vi "Panel.vi"(11 "SimpleGraphEditorPanel in":refnum<class "SimpleGraphEditorPanel.lvclass">) -> ()   [LabVIEW 2020, in "VolatusGUIControls.lvlib" / "SimpleGraphEditorPanel.lvclass"]
uses:
  SimpleGraphEditorPanel.lvclass
  C:/dev/lv20CE/relink/volatus-gui-controls/VolatusGUIEditorCore/ElementEditorPanel/ElementEditorPanel.lvclass
  C:/dev/lv20CE/relink/lv-oopanel/OOPanel/Panel/Panel.lvclass
  lv-oopanel/OOPanel/Panel/Basic UI State.ctl
  SimpleGraphEditorPanel.lvclass/SimpleGraphEditorPanel.ctl
  lv-autocomplete/AutoComplete/Shared Options/Shared Options.lvclass/Shared Options.ctl
  lv-oopanel/OOPanel/Panel/Panel.lvclass
  lv-oopanel/OOPanel/OOPanel.lvlib
  VolatusGUIEditorCore/ElementEditorPanel/ElementEditorPanel.lvclass
  VolatusGUIEditorCore/VolatusGUIEditorCore.lvlib
  C:/dev/lv20CE/relink/volatus-gui-controls/VolatusGUIControls/SimpleGraphEditorPanel/SimpleGraphEditorPanel.lvclass
panel:
  in  "Legend Scrollbar":bool
  in  "Plot Visibility Checkbox":bool
  in  "Show Legend":bool
  in  "History Minutes":dbl
  in  "Scales":bool
  in  "Channels":bool
  in  "Top":i32
  in  "Left":i32
  in  "Height":u16
  in  "Width":u16
  in  "Label Text Color":u32(colorbox) caption="Color"
  in  "Label Visible":bool caption="Visible"
  in  "Label":string
  # "Label"
  # "Assumes 10Hz published data"
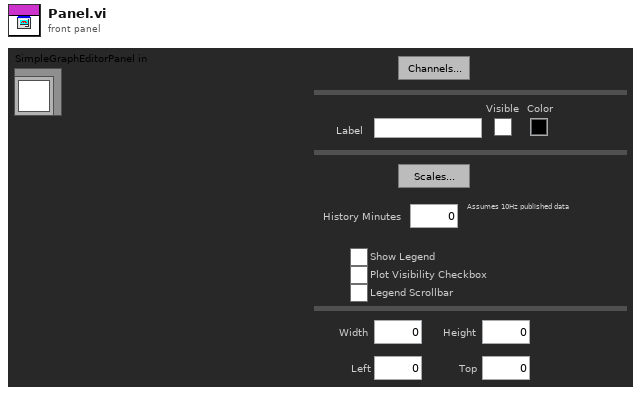
[diagram p1: front panel]
types:
  T1 = typedef "OOPanel.lvlib/Panel.lvclass/Basic UI State.ctl" = enum16{"Init", "Run", "Close"}
  T2 = typedef "VolatusGUIEditorCore.lvlib/ElementEditorPanel.lvclass/Incoming Events.ctl" = cluster{"Update Control":refnum<user-event>}
  T3 = typedef "OOPanel.lvlib/Panel.lvclass/Panel Events.ctl" = cluster{"Visbility":refnum<user-event>, "Close":refnum<user-event>}
  T4 = typedef "VolatusGUIControls.lvlib/SimpleGraphEditorPanel.lvclass/Props.ctl" = cluster{"JSON Props":T5, "Label":T6, "Position":T7, "Width":u16, "Height":u16, "Plot Legend":T8}
  T5 = typedef "VolatusGUIControls.lvlib/SimpleGraphEditorPanel.lvclass/JSON Props.ctl" = cluster{"Channels":string[], "Buffer_Length":i32, "Redraw_Period_s":dbl, "Duration_s":i32}
  T6 = typedef "VolatusGUIEditorCore.lvlib/Label Props.ctl" = cluster{"Text":string, "Text Color":u32, "Visible":bool}
  T7 = typedef "VolatusGUIEditorCore.lvlib/Position Props.ctl" = cluster{"Left":i32, "Top":i32}
  T8 = typedef "VolatusGUIEditorCore.lvlib/Plot Legend Props.ctl" = cluster{"Visible":bool, "Plot Visibility":bool, "Scrollbar":bool}
  T9 = typedef "OOPanel.lvlib/Visibility State.ctl" = enum16{"Idle", "Closed", "Hidden", "Visible", "Subpanel", "Hidden Subpanel"}
  T10 = cluster{"Label":string, "Label Text Color":u32, "Label Visible":bool}
  T11 = cluster{"Show Legend":bool, "Plot Visibility Checkbox":bool, "Legend Scrollbar":bool}
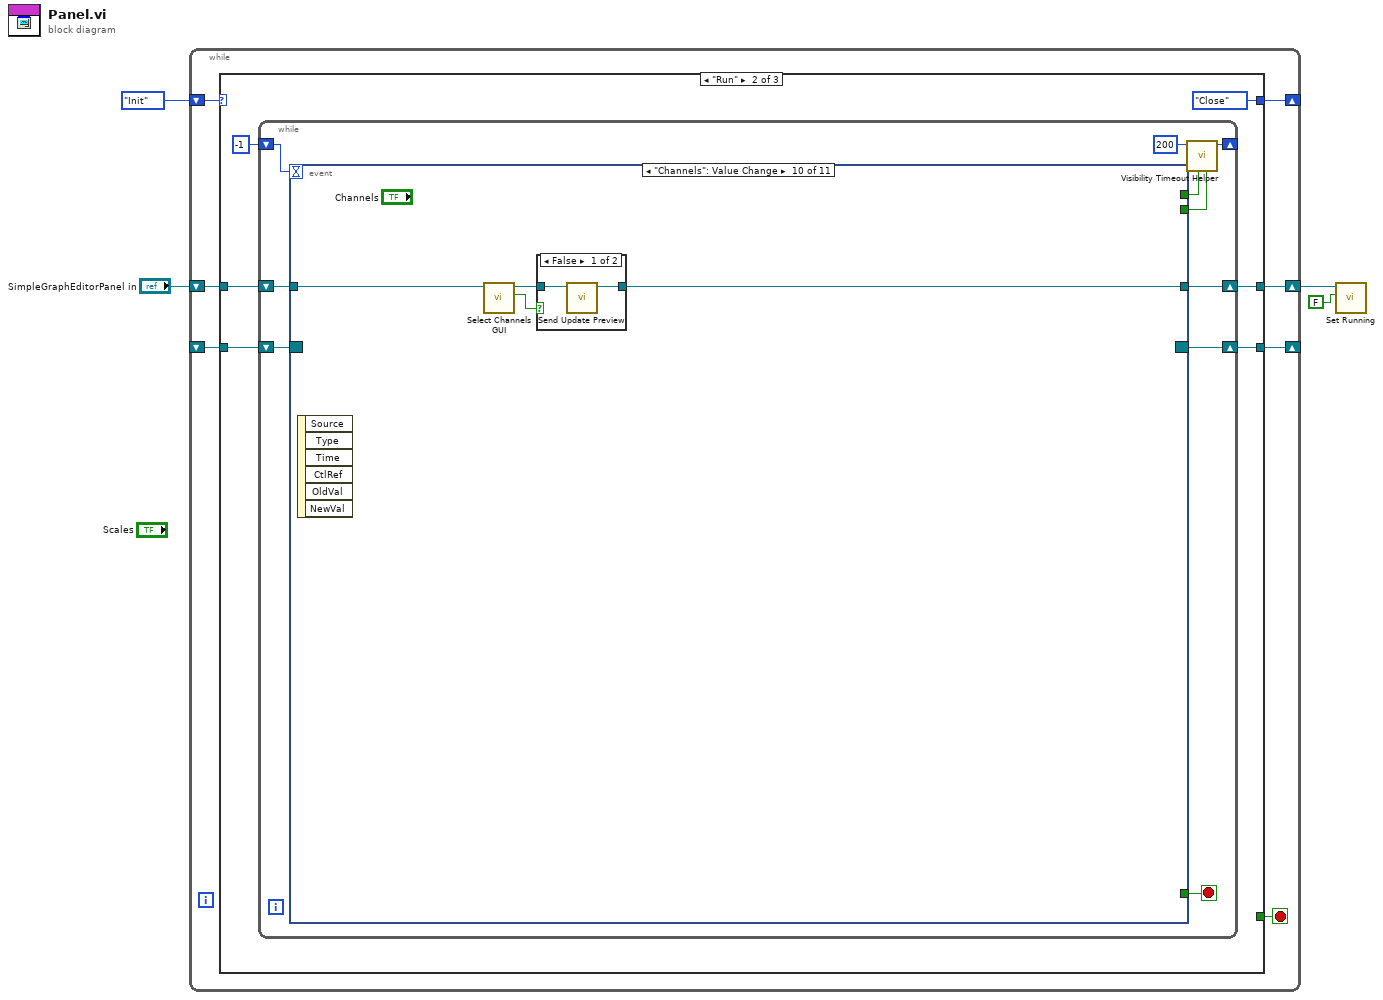
[diagram p0: block diagram]
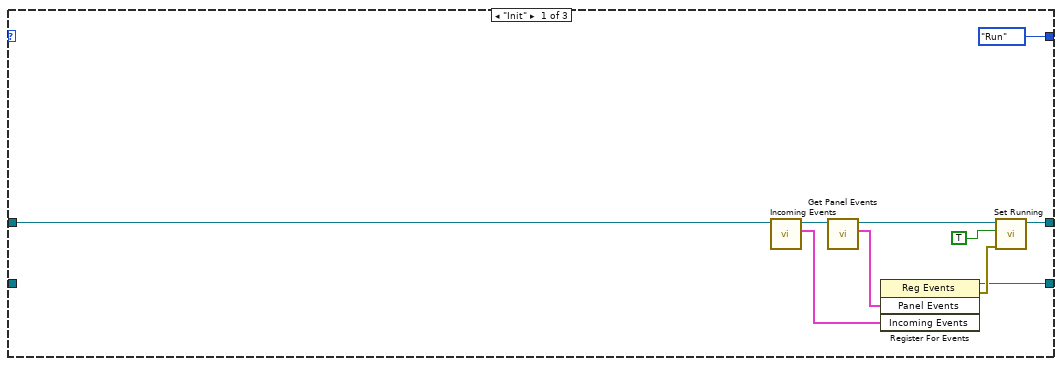
[diagram p2: hidden frame]
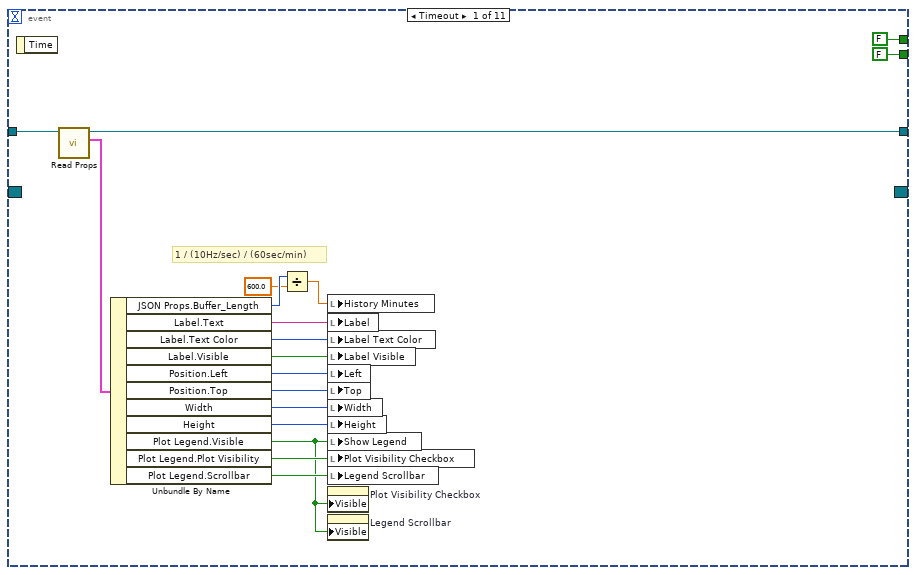
[diagram p3: hidden frame]
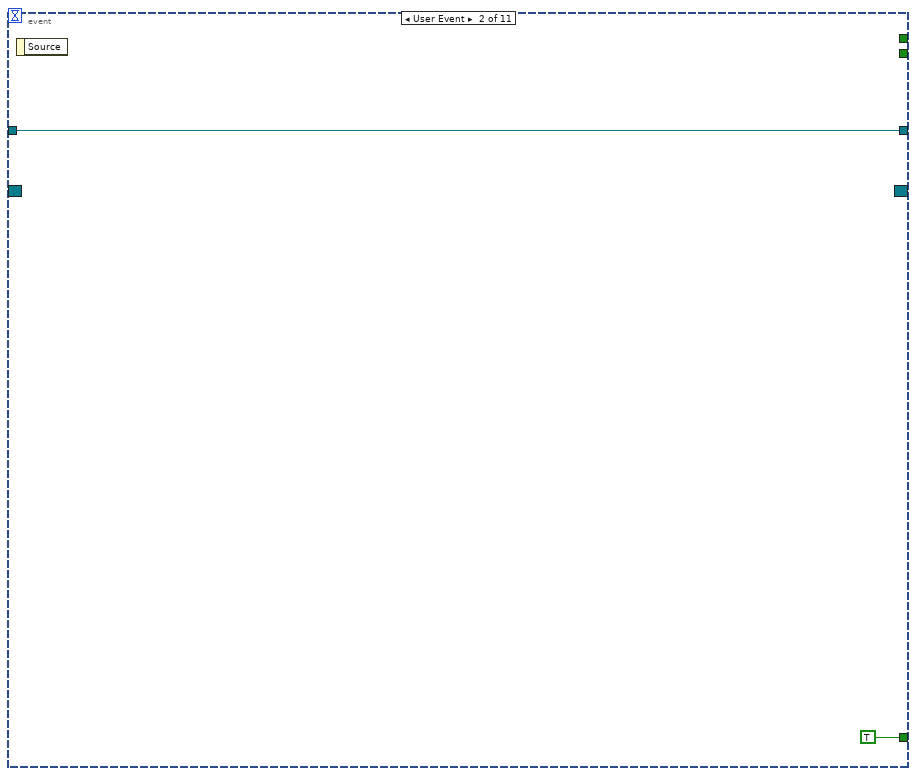
[diagram p4: hidden frame]
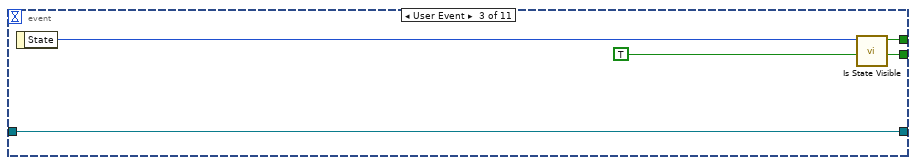
[diagram p5: hidden frame]
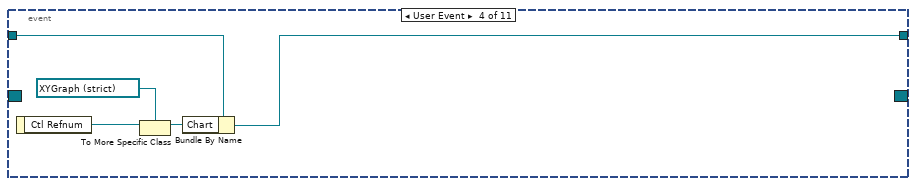
[diagram p6: hidden frame]
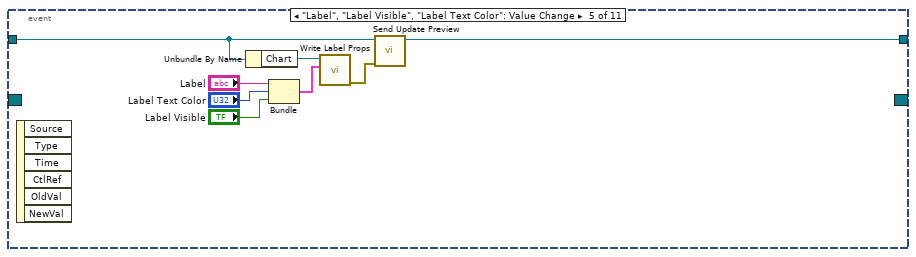
[diagram p7: hidden frame]
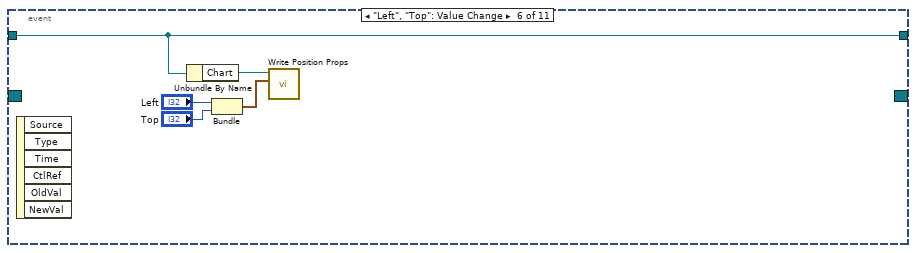
[diagram p8: hidden frame]
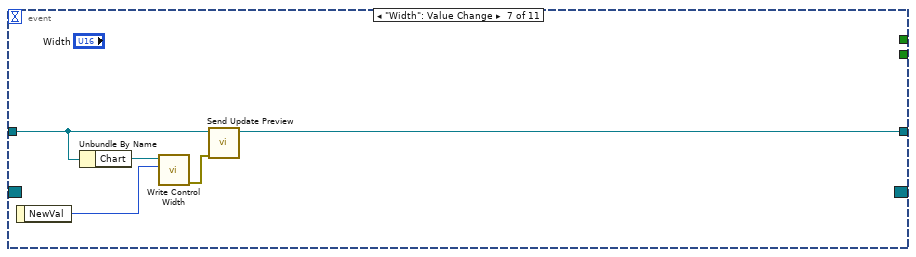
[diagram p9: hidden frame]
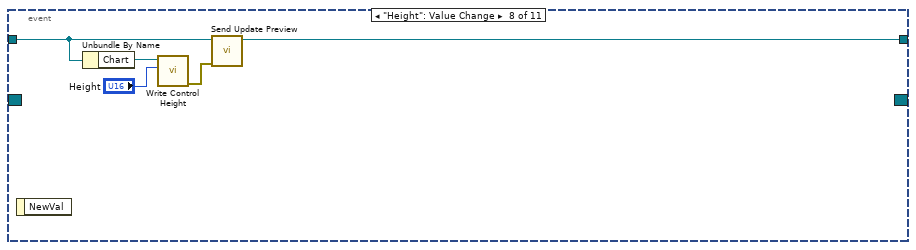
[diagram p10: hidden frame]
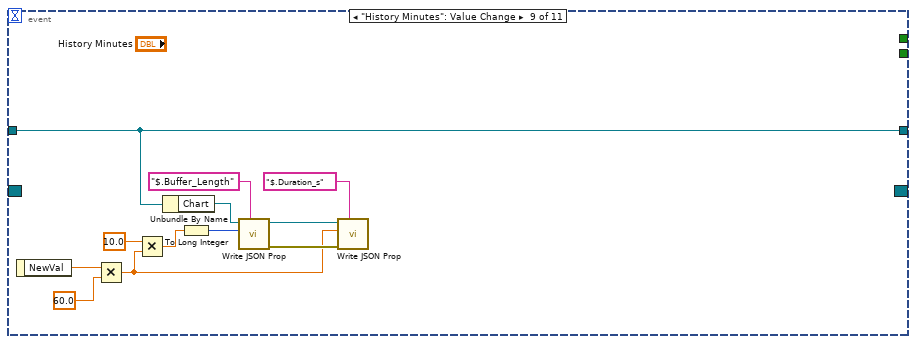
[diagram p11: hidden frame]
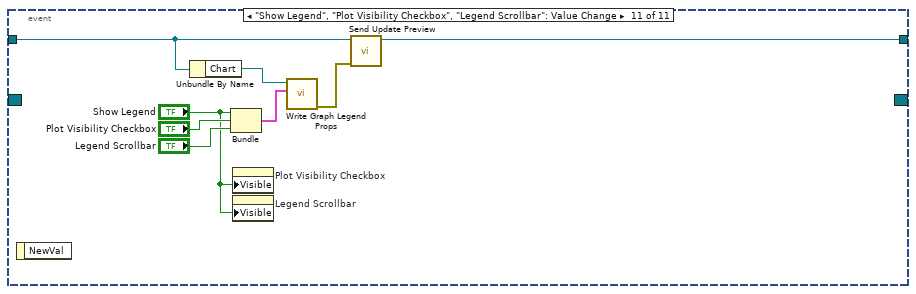
[diagram p13: hidden frame]
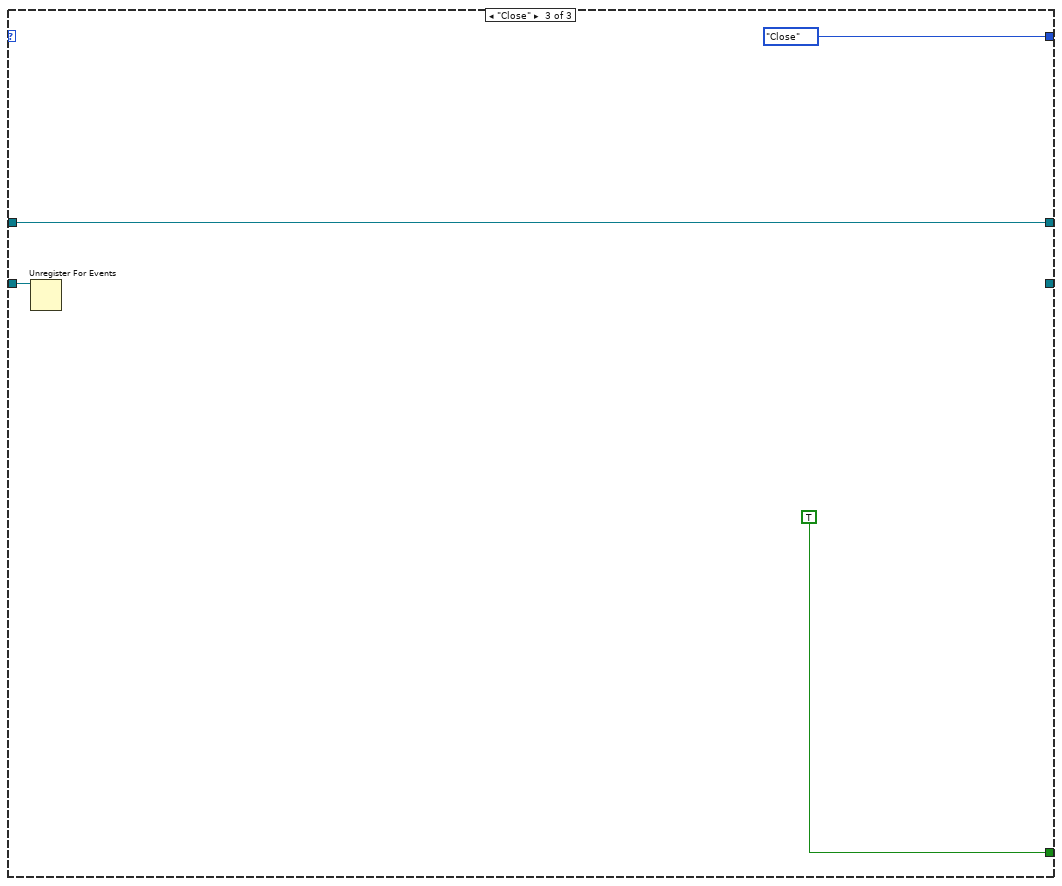
[diagram p14: hidden frame]
diagram:
  n1 = while {
    shift-right: [w10] -> _
    shift-left: _ -> [w11]
    shift-right: [w8] -> _
    shift-left: Basic_UI_State."Init" ("Basic UI State") -> [w9]
    shift-right: [w6] -> w4
    shift-left: "SimpleGraphEditorPanel in" -> [w5]
    stop <- w7 stop-if-true
    n2 = case shown="\"Run\"" w9 {
      tunnel: w11 -> [_ w27 w118]
      tunnel: [w18 w25 _] -> w10
      tunnel: [Basic_UI_State."Run" ("Basic UI State") Basic_UI_State."Close" ("Basic UI State") Basic_UI_State."Close" ("Basic UI State")] -> w8
      tunnel: [_ _ TRUE] -> w7
      tunnel: [w17 w22 w117] -> w6
      tunnel: w5 -> [w16 w23 w117]
      frame "Init" {
        n3 = call "Incoming Events.vi"("ElementEditorPanel in"=w16) -> ("Incoming Events"=w12:T2, "ElementEditorPanel out"=w13:refnum<class "SimpleGraphEditorPanel.lvclass">)  [unwired: 9 in]
        n4 = call "Get Panel Events.vi"("Panel in"=w13) -> ("Panel Events"=w14:T3, "Panel out"=w15:refnum<class "SimpleGraphEditorPanel.lvclass">)  [unwired: 8 in, 1 out]
        n5 = register-events(w14, w12) -> (reference out=w18:refnum<event-registration>, error out=w20:errorcluster)  [unwired: 2 in]
        n6 = call "Set Running.vi"("error in (no error)"=w20, "Running"=TRUE, "Panel in"=w15) -> ("Panel out"=w17:refnum<class "SimpleGraphEditorPanel.lvclass">)  [unwired: 7 in, 1 out]
      }
      frame "Run" {
        n7 = while {
          shift-right: [w33] -> w25
          shift-left: w27 -> [w34]
          shift-right: [w36] -> _
          shift-left: -1 ("Timeout") -> [w35]
          shift-right: [w28] -> w22
          shift-left: w23 -> [w29]
          stop <- w30 stop-if-true
          n8 = event shown="[9] \"Channels\": Value Change" {
            selector: w34 -> [_ _ _ _ _ _ _ _ _ _ _]
            dyn-events: [_ _ _ _ _ _ _ _ _ _ _] -> w33
            timeout: w35 -> [_ _ _ _ _ _ _ _ _ _ _]
            tunnel: [FALSE _ w60 _ _ _ _ _ _ _ _] -> w32
            tunnel: [FALSE _ TRUE _ _ _ _ _ _ _ _] -> w31
            tunnel: [_ TRUE _ _ _ _ _ _ _ _ _] -> w30
            tunnel: w29 -> [w53 w56 w58 w66 w72 w76 w84 w88 w97 w102 w116]
            tunnel: [w52 w56 w58 w64 w68 w76 w81 w86 w97 w104 w111] -> w28
            event Timeout {
              # "1 / (10Hz/sec) / (60sec/min)"
              n9 = event-data() -> ()  [unwired: 1 in, 1 out]
              n10 = call "Read Props.vi"("SimpleGraphEditorPanel in"=w53) -> ("Props"=w51:T4, "SimpleGraphEditorPanel out"=w52:refnum<class "SimpleGraphEditorPanel.lvclass">)  [unwired: 8 in, 1 out]
              n11 = Unbundle By Name(w51) -> ("JSON Props.Buffer_Length"=w50:i32, "Label.Text"=w48:string, "Label.Text Color"=w47:u32, "Label.Visible"=w46:bool, "Position.Left"=w45:i32, "Position.Top"=w44:i32, "Width"=w43:u16, "Height"=w42:u16, "Plot Legend.Visible"=w38:bool, "Plot Legend.Plot Visibility"=w40:bool, "Plot Legend.Scrollbar"=w39:bool)
              n12 = Divide(x=w50, y=600.0) -> (x/y=w41:dbl)
              n13 = local write "History Minutes"(w41) -> ()
              n14 = local write "Label"(w48) -> ()
              n15 = local write "Label Text Color"(w47) -> ()
              n16 = local write "Label Visible"(w46) -> ()
              n17 = local write "Left"(w45) -> ()
              n18 = local write "Top"(w44) -> ()
              n19 = local write "Width"(w43) -> ()
              n20 = local write "Height"(w42) -> ()
              n21 = local write "Show Legend"(w38) -> ()
              n22 = local write "Plot Visibility Checkbox"(w40) -> ()
              n23 = local write "Legend Scrollbar"(w39) -> ()
              n24 = property on="Plot Visibility Checkbox" class="Bool (strict)"("Visible"=w38) -> ()  [unwired: 2 in, 2 out]
              n25 = property on="Legend Scrollbar" class="Bool (strict)"("Visible"=w38) -> ()  [unwired: 2 in, 2 out]
            }
            event User Event {
              n26 = event-data() -> ()  [unwired: 1 in, 1 out]
            }
            event User Event {
              n27 = event-data() -> ("State"=w61:T9)  [unwired: 1 in]
              n28 = call "Is State Visible.vi"("Visibility"=w61) -> ("Visible"=w60:bool)  [unwired: 10 in]
            }
            event User Event {
              n29 = event-data() -> ("Ctl Refnum"=w65:refnum<vi>)  [unwired: 1 in]
              n30 = To More Specific Class(target class=refnum<vi> refnum ("Chart"), reference=w65) -> (specific class reference=w62:refnum<vi>)  [unwired: 1 in, 1 out]
              n31 = Bundle By Name(cluster=w66, "Chart"=w62) -> (w64:refnum<class "SimpleGraphEditorPanel.lvclass">)
            }
            event "Label", "Label Visible", "Label Text Color": Value Change {
              n32 = event-data() -> ()  [unwired: 1 in, 6 out]
              n33 = Unbundle By Name(w72) -> ("Chart"=w69:refnum<vi>)
              n34 = Bundle("Label"="Label", "Label Text Color"="Label Text Color", "Label Visible"="Label Visible") -> (w73:T10)  [unwired: 1 in]
              n35 = call "Write Label Props.vi"("Label Props"=w73, "Ctl Refnum in"=w69) -> ("error out"=w67:errorcluster)  [unwired: 8 in, 1 out]
              n36 = call "Send Update Preview.vi"("error in (no error)"=w67, "ElementEditorPanel in"=w72) -> ("ElementEditorPanel out"=w68:refnum<class "SimpleGraphEditorPanel.lvclass">)  [unwired: 8 in, 1 out]
            }
            event "Left", "Top": Value Change {
              n37 = event-data() -> ()  [unwired: 1 in, 6 out]
              n38 = Unbundle By Name(w76) -> ("Chart"=w75:refnum<vi>)
              n39 = Bundle("Left"="Left", "Top"="Top") -> (w77:cluster{"Left":i32, "Top":i32})  [unwired: 1 in]
              n40 = call "Write Position Props.vi"("Position Props"=w77, "Ctl Refnum in"=w75) -> ()  [unwired: 8 in, 2 out]
            }
            event "Width": Value Change {
              n41 = event-data() -> ("NewVal"=w82:u16)  [unwired: 1 in]
              n42 = Unbundle By Name(w84) -> ("Chart"=w83:refnum<vi>)
              n43 = call "Write Control Width.vi"("Width"=w82, "Control in"=w83) -> ("error out"=w80:errorcluster)  [unwired: 8 in, 1 out]
              n44 = call "Send Update Preview.vi"("error in (no error)"=w80, "ElementEditorPanel in"=w84) -> ("ElementEditorPanel out"=w81:refnum<class "SimpleGraphEditorPanel.lvclass">)  [unwired: 8 in, 1 out]
            }
            event "Height": Value Change {
              n45 = event-data() -> ()  [unwired: 1 in, 1 out]
              n46 = Unbundle By Name(w88) -> ("Chart"=w87:refnum<vi>)
              n47 = call "Write Control Height.vi"("Height"="Height", "Control in"=w87) -> ("error out"=w85:errorcluster)  [unwired: 8 in, 1 out]
              n48 = call "Send Update Preview.vi"("error in (no error)"=w85, "ElementEditorPanel in"=w88) -> ("ElementEditorPanel out"=w86:refnum<class "SimpleGraphEditorPanel.lvclass">)  [unwired: 8 in, 1 out]
            }
            event "History Minutes": Value Change {
              n49 = event-data() -> ("NewVal"=w101:dbl)  [unwired: 1 in]
              n50 = Multiply(x=w101, y=60.0) -> (x*y=w90:dbl)
              n51 = Multiply(x=10.0, y=w90) -> (x*y=w94:dbl)
              n52 = Unbundle By Name(w97) -> ("Chart"=w99:refnum<vi>)
              n53 = To Long Integer(number=w94) -> (32bit integer=w96:i32)
              n54 = call "Write JSON Prop.vi"("JSON Path"="$.Buffer_Length" ("$Path or Item Name"), "Value"=w96, "Ctl Refnum in"=w99) -> ("error out"=w92:errorcluster, "Ctl Refnum"=w93:refnum<vi>)  [unwired: 7 in]
              n55 = call "Write JSON Prop.vi"("JSON Path"="$.Duration_s" ("$Path or Item Name"), "error in (no error)"=w92, "Value"=w90, "Ctl Refnum in"=w93) -> ()  [unwired: 6 in, 2 out]
            }
            event "Channels": Value Change {
              n56 = event-data() -> ()  [unwired: 1 in, 6 out]
              n57 = call "Select Channels GUI.vi"("SimpleGraphEditorPanel in"=w102) -> ("Cancelled"=w103:bool, "SimpleGraphEditorPanel out"=w105:refnum<class "SimpleGraphEditorPanel.lvclass">)  [unwired: 8 in, 1 out]
              n58 = case shown="False" w103 {
                tunnel: w105 -> [w107 w108]
                tunnel: [w106 w108] -> w104
                frame False {
                  n59 = call "Send Update Preview.vi"("ElementEditorPanel in"=w107) -> ("ElementEditorPanel out"=w106:refnum<class "SimpleGraphEditorPanel.lvclass">)  [unwired: 9 in, 1 out]
                }
                frame True {
                }
              }
            }
            event "Show Legend", "Plot Visibility Checkbox", "Legend Scrollbar": Value Change {
              n60 = event-data() -> ()  [unwired: 1 in, 1 out]
              n61 = Unbundle By Name(w116) -> ("Chart"=w112:refnum<vi>)
              n62 = Bundle("Show Legend"="Show Legend", "Plot Visibility Checkbox"="Plot Visibility Checkbox", "Legend Scrollbar"="Legend Scrollbar") -> (w113:T11)  [unwired: 1 in]
              n63 = property on="Plot Visibility Checkbox" class="Bool (strict)"("Visible"="Show Legend") -> ()  [unwired: 2 in, 2 out]
              n64 = property on="Legend Scrollbar" class="Bool (strict)"("Visible"="Show Legend") -> ()  [unwired: 2 in, 2 out]
              n65 = call "Write Graph Legend Props.vi"("Plot Legend Props"=w113, "Graph in"=w112) -> ("error out"=w110:errorcluster)  [unwired: 8 in, 1 out]
              n66 = call "Send Update Preview.vi"("error in (no error)"=w110, "ElementEditorPanel in"=w116) -> ("ElementEditorPanel out"=w111:refnum<class "SimpleGraphEditorPanel.lvclass">)  [unwired: 8 in, 1 out]
            }
          }
          n67 = call "Visibility Timeout Helper.vi"("Update?"=w31, "Use Timeout?"=w32, "Visible Timeout mS"=200) -> ("Timeout"=w36:i32)  [unwired: 8 in]
        }
      }
      frame "Close" {
        n68 = Unregister For Events(event registration refnum=w118) -> ()  [unwired: 1 in, 1 out]
      }
    }
  }
  n69 = call "Set Running.vi"("Running"=FALSE, "Panel in"=w4) -> ()  [unwired: 8 in, 2 out]
